vi "TEST.vi"() -> ()   [LabVIEW 2019]
panel:
  out "t0":dbl
  out "t1":dbl
  out "Array 2":dbl[][](array[numeric])
  out "Array":dbl[][](array[numeric])
  out "text":string
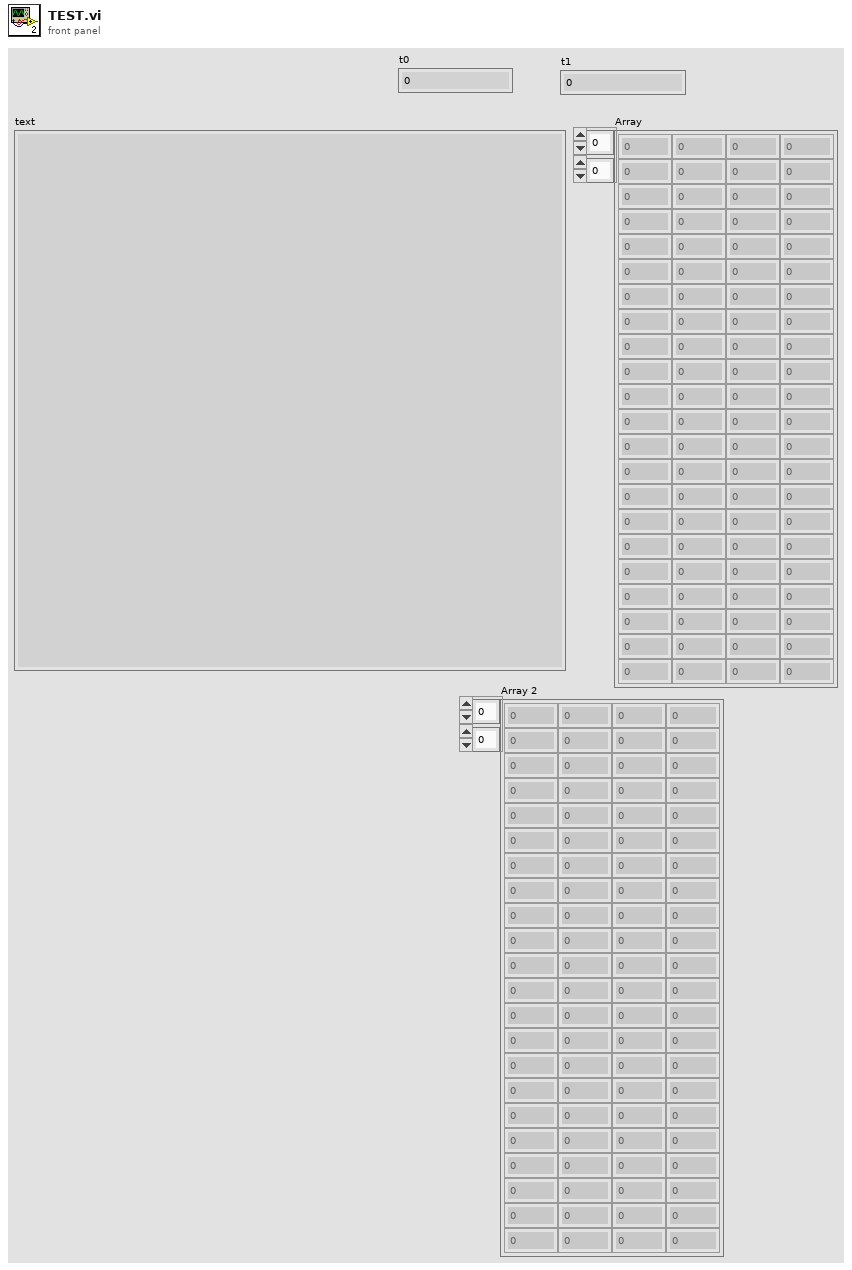
[diagram p1: front panel]
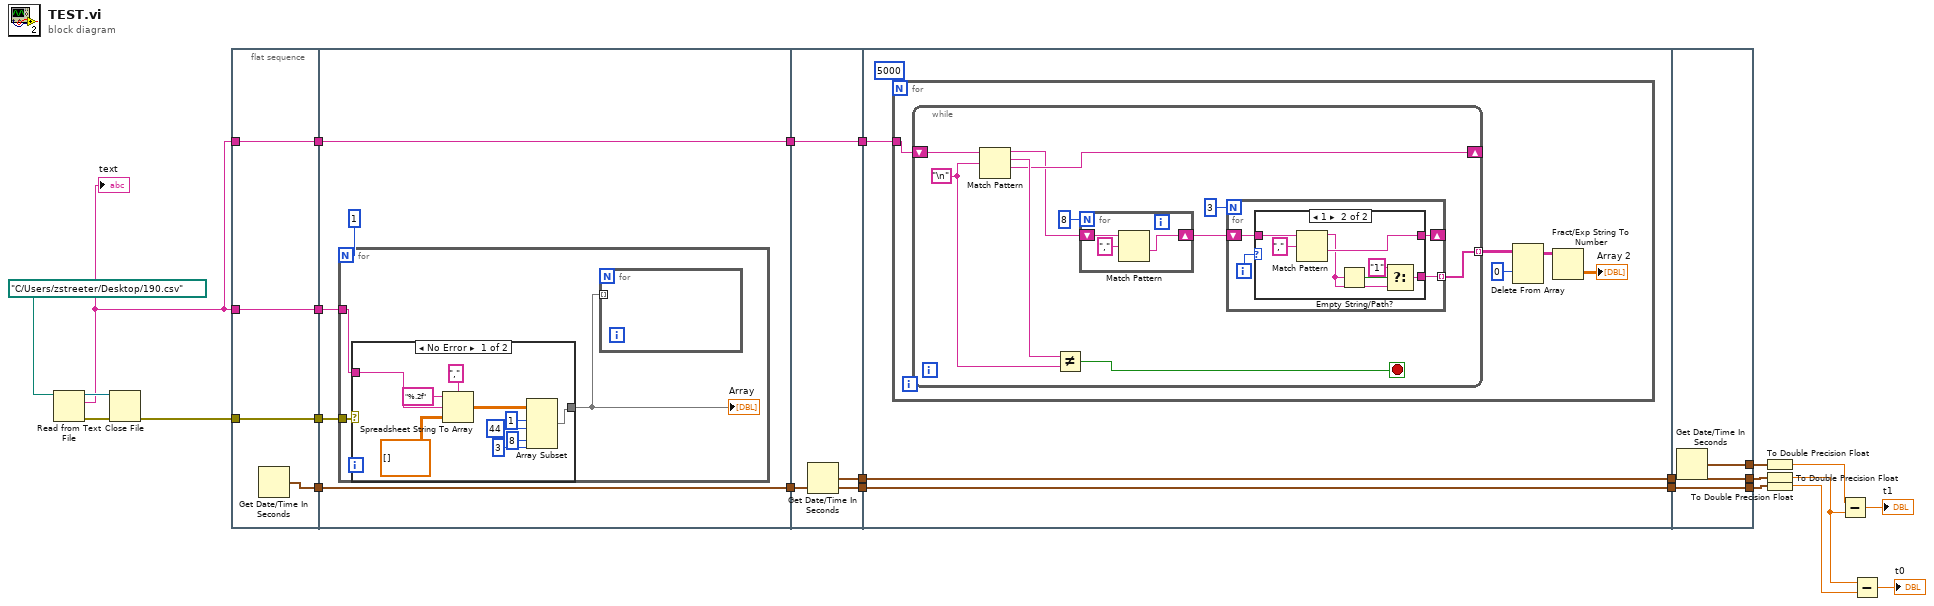
[diagram p0: block diagram]
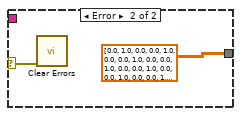
[diagram p2: hidden frame]
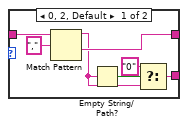
[diagram p3: hidden frame]
diagram:
  n1 = Read from Text File(file (use dialog)=path "C:/Users/zstreeter/Desktop/190.csv" ("Path")) -> (refnum out=w21:refnum<file>, text=w9:string, error out=w22:errorcluster)  [unwired: 3 in, 1 out]
  "text" <- w9
  n2 = Close File(refnum=w21, error in=w22) -> (error out=w24:errorcluster)  [unwired: 1 out]
  n3 = flat-sequence {
    tunnel: w9 -> [w27]
    tunnel: w24 -> [w28]
    tunnel: [w28] -> w20
    tunnel: [w27] -> w19
    tunnel: [w26] -> w17
    tunnel: [w25] -> w10
    tunnel: w9 -> [w25]
    tunnel: w20 -> [w33]
    tunnel: w19 -> [w32]
    tunnel: [w31] -> w18
    tunnel: w17 -> [w31]
    tunnel: [w30] -> w11
    tunnel: w10 -> [w30]
    tunnel: w18 -> [w50]
    tunnel: [w51] -> w14
    tunnel: [w50] -> w13
    tunnel: [w49] -> w12
    tunnel: w11 -> [w49]
    tunnel: w14 -> [w55]
    tunnel: w13 -> [w54]
    tunnel: w12 -> [w53]
    tunnel: [w55] -> w8
    tunnel: [w54] -> w7
    tunnel: [w93] -> w6
    tunnel: [w94] -> w5
    tunnel: w8 -> [w94]
    tunnel: w7 -> [w93]
    tunnel: [w92] -> w4
    frame #0 {
      n4 = Get Date/Time In Seconds() -> (seconds since 1Jan1904=w26:timestamp)
    }
    frame #1 {
      n5 = for {
        N: 1 -> [_]
        tunnel: w33 -> [w36]
        tunnel: w32 -> [w35]
        n6 = case shown="No Error" w36 {
          selector: w36 -> [_ w48]
          tunnel: w35 -> [w44 _]
          tunnel: [w41 dbl[][] [[0.0, 1.0, 0.0], [0.0, 1.0, 0.0], [0.0, 1.0, 0.0], [0.0, 1.0, 0.0], [0.0, 1.0, 0.0], [0.0, 1.0, 0.0], [0.0, 1.0, 0.0], [0.0, 1.0, 0.0], [0.0, 1.0, 0.0], [0.0, 1.0, 0.0], [0.0, 1.0, 0.0], [0.0, 1.0, 0.0], [0.0, 1.0, 0.0], [0.0, 1.0, 0.0], [0.0, 1.0, 0.0], [0.0, 1.0, 0.0], [0.0, 1.0, 0.0], [0.0, 1.0, 0.0], [0.0, 1.0, 0.0], [0.0, 1.0, 0.0], [0.0, 1.0, 0.0], [0.0, 1.0, 0.0], [0.0, 1.0, 0.0], [0.0, 1.0, 0.0], [0.0, 1.0, 0.0], [0.0, 1.0, 0.0], [0.0, 1.0, 0.0], [0.0, 1.0, 0.0], [0.0, 1.0, 0.0], [0.0, 1.0, 0.0], [0.0, 1.0, 0.0], [0.0, 1.0, 0.0], [0.0, 1.0, 0.0], [0.0, 1.0, 0.0], [0.0, 1.0, 0.0], [0.0, 1.0, 0.0], [0.0, 1.0, 0.0], [0.0, 1.0, 0.0], [0.0, 1.0, 0.0], [0.0, 1.0, 0.0], [0.0, 1.0, 0.0], [0.0, 1.0, 0.0], [0.0, 1.0, 0.0], [0.0, 1.0, 0.0]]] -> w34
          frame No Error {
            n7 = Spreadsheet String To Array(delimiter (Tab)=",", format string="%.2f", spreadsheet string=w44, array type (2D Dbl)=dbl[][] []) -> (array=w42:dbl[][])
            n8 = Array Subset(array=w42, index (row)=1 ("index"), length (row)=44 ("length"), index (col)=8 ("index"), length (col)=3 ("length")) -> (w41:dbl[][])
          }
          frame Error {
            n9 = call <vilib>:"Clear Errors.vi"("error in (no error)"=w48) -> ()  [unwired: 5 in, 2 out]
          }
        }
        "Array" <- w34
        n10 = for {
          tunnel: w34 -> [_] mode=indexing
        }
      }
    }
    frame #2 {
      n11 = Get Date/Time In Seconds() -> (seconds since 1Jan1904=w51:timestamp)
    }
    frame #3 {
      n12 = for {
        N: 5000 -> [_]
        tunnel: w53 -> [w60]
        n13 = while {
          shift-right: [w66] -> _
          shift-left: w60 -> [w70]
          tunnel: [w61] -> w58 mode=indexing
          stop <- w67 stop-if-true
          w68 = "\n"
          n14 = Match Pattern(string=w70, regular expression=w68) -> (before substring=w62:string, match substring=w69:string, after substring=w66:string)  [unwired: 1 in, 1 out]
          n15 = Not Equal?(x=w69, y=w68) -> (x != y?=w67:bool)
          n16 = for {
            N: 8 -> [_]
            shift-right: [w71] -> w65
            shift-left: w62 -> [w72]
            n17 = Match Pattern(string=w72, regular expression=",") -> (after substring=w71:string)  [unwired: 1 in, 3 out]
          }
          n18 = for {
            N: 3 -> [_]
            shift-right: [w75] -> _
            shift-left: w65 -> [w76]
            tunnel: [w74] -> w61 mode=indexing
            i -> [w77]
            n19 = case shown="1" w77 {
              tunnel: w76 -> [w84 w91]
              tunnel: [w83 w90] -> w75
              tunnel: [w78 w85] -> w74
              frame 0, 2, Default {
                n20 = Match Pattern(string=w84, regular expression=",") -> (before substring=w79:string, after substring=w83:string)  [unwired: 1 in, 2 out]
                n21 = Empty String/Path?(string/path=w79) -> (empty?=w81:bool)
                n22 = Select(t="0", s=w81, f=w79) -> (s? t:f=w78:string)
              }
              frame 1 {
                n23 = Match Pattern(string=w91, regular expression=",") -> (before substring=w87:string, after substring=w90:string)  [unwired: 1 in, 2 out]
                n24 = Empty String/Path?(string/path=w87) -> (empty?=w88:bool)
                n25 = Select(t="1", s=w88, f=w87) -> (s? t:f=w85:string)
              }
            }
          }
        }
        n26 = Delete From Array(array=w58, index (row)=0) -> (array with subset deleted=w57:string[][])  [unwired: 2 in, 1 out]
        n27 = Fract/Exp String To Number(string=w57) -> (number=→"Array 2":dbl[][])  [unwired: 3 in, 1 out]
      }
    }
    frame #4 {
      n28 = Get Date/Time In Seconds() -> (seconds since 1Jan1904=w92:timestamp)
    }
  }
  n29 = To Double Precision Float(number=w4) -> (double precision float=w1:dbl)
  n30 = To Double Precision Float(number=w5) -> (double precision float=w2:dbl)
  n31 = To Double Precision Float(number=w6) -> (double precision float=w3:dbl)
  n32 = Subtract(x=w1, y=w2) -> (x-y=→"t1":dbl)
  n33 = Subtract(x=w2, y=w3) -> (x-y=→"t0":dbl)
